vi "GetLibraryDependencies.vi"(11 "FileDependency":map{path, T1}(c390)) -> (2 "LibraryDependency":map{path, T3}(c390))   [LabVIEW 2020, in "DependencyViewer.lvlib"]
uses:
  DependencyViewer/DependencyViewer.lvlib
  LibraryDependentInfo.vi
  <vilib>/Utility/lvfile.llb/FT_FileTypes.ctl
  FileDependencyType.ctl
  <vilib>/Utility/miscctls.llb/LVMapReplaceAction.ctl
  <vilib>/Utility/lvfile.llb/NI_FileType.lvlib
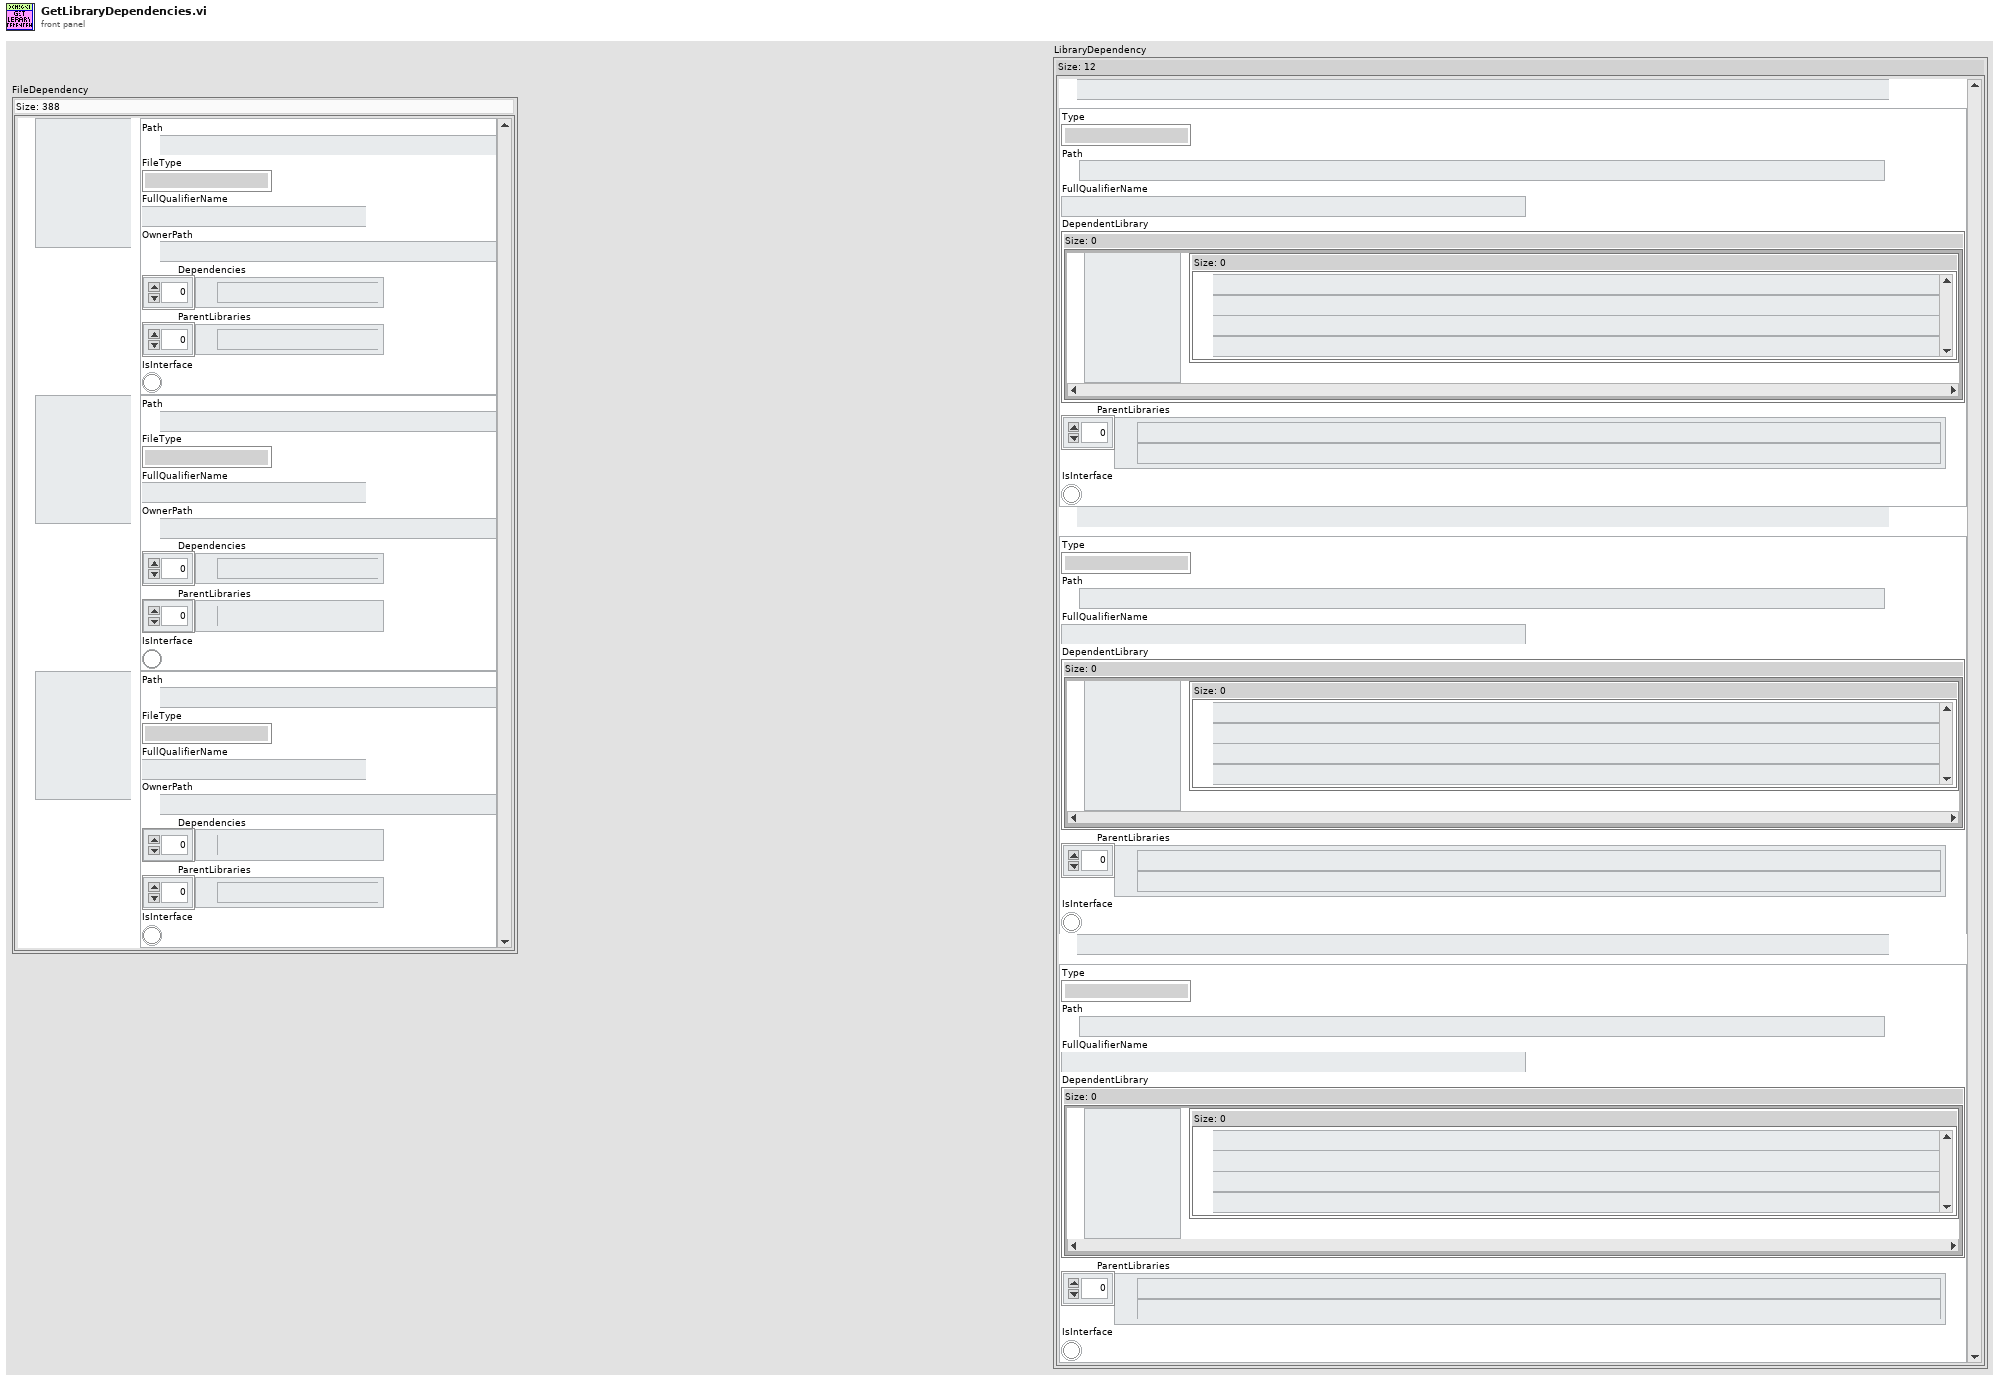
[diagram p1: front panel]
types:
  T1 = typedef "DependencyViewer.lvlib/FileDependencyType.ctl" = cluster{"Path":path, "FileType":T2, "FullQualifierName":string, "OwnerPath":path, "Dependencies":path[], "ParentLibraries":path[], "IsInterface":bool}
  T2 = typedef "NI_FileType.lvlib/FT_FileTypes.ctl" = enum32{"Invalid file/path", "Unknown type", "Instrument", "Control", "Polymorphic VI", "Project", "Library", "LVClass", "XControl", "XNode", "CIN", "Run-time menu", "Palette menu", "LLB", "Shortcut", "Directory", "Class Private Data Control", "Statechart", "MathScript .m file", "Ladder Diagram", "LVLibp"}
  T3 = typedef "DependencyViewer.lvlib/LibraryDependentInfo.vi" = cluster{"Type":T2, "Path":path, "FullQualifierName":string, "DependentLibrary":map{path, set{path}}, "ParentLibraries":path[], "IsInterface":bool}
  T4 = typedef "LVMapReplaceAction.ctl" = enum32{"Modify Entry only if found", "Add or Modify Entry", "Delete Entry"}
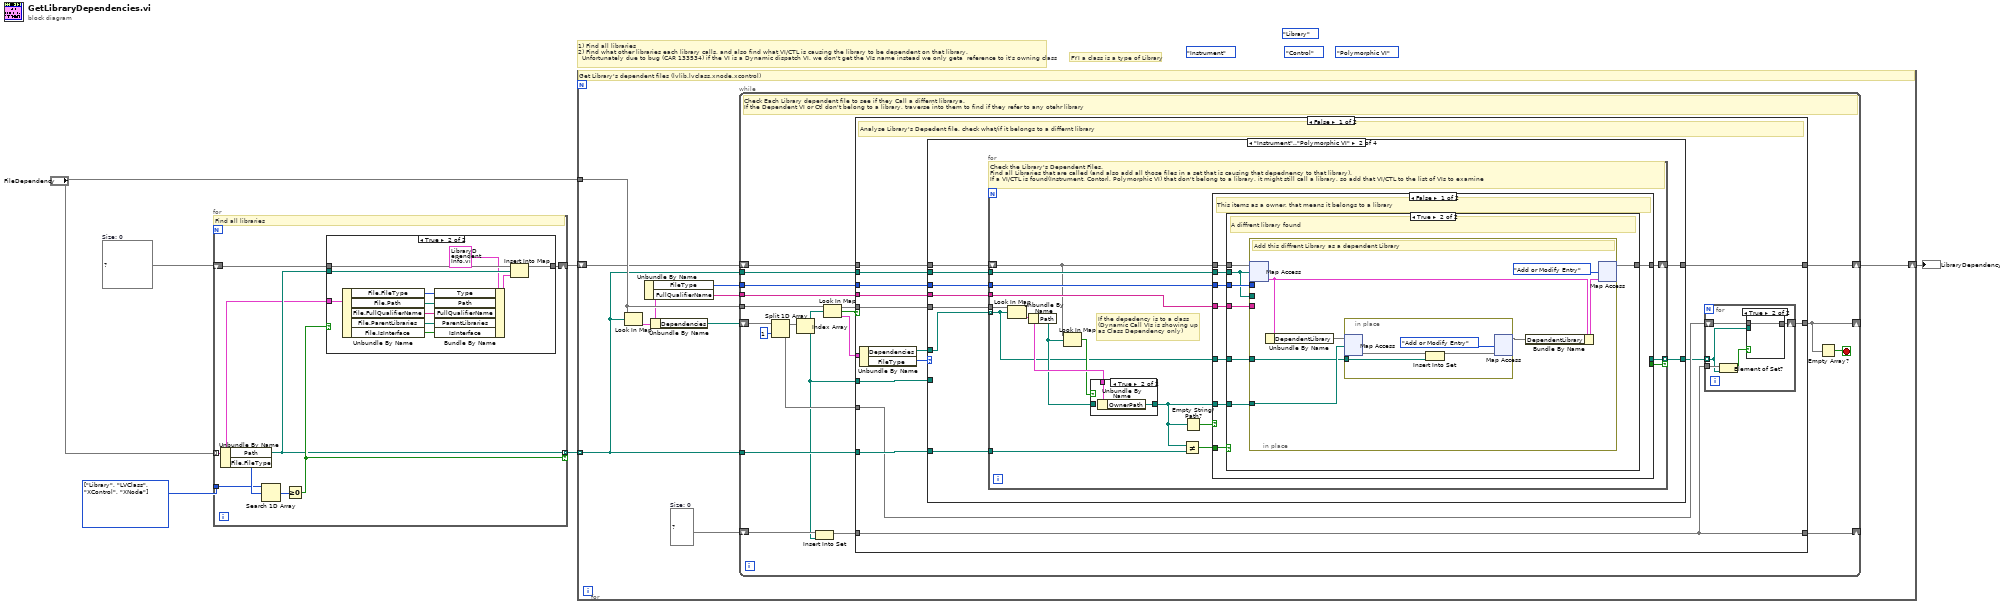
[diagram p0: block diagram]
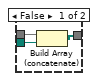
[diagram p2: hidden frame]
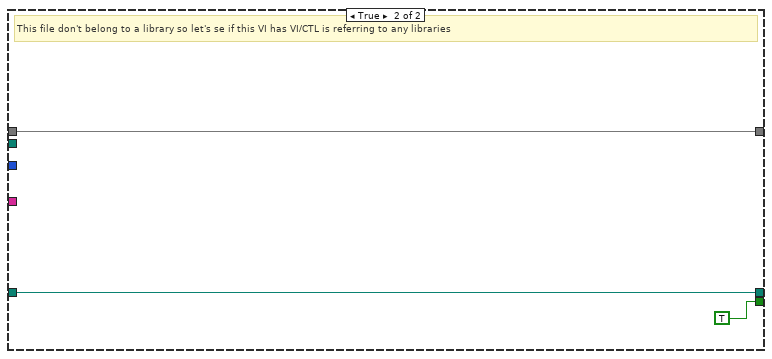
[diagram p5: hidden frame]
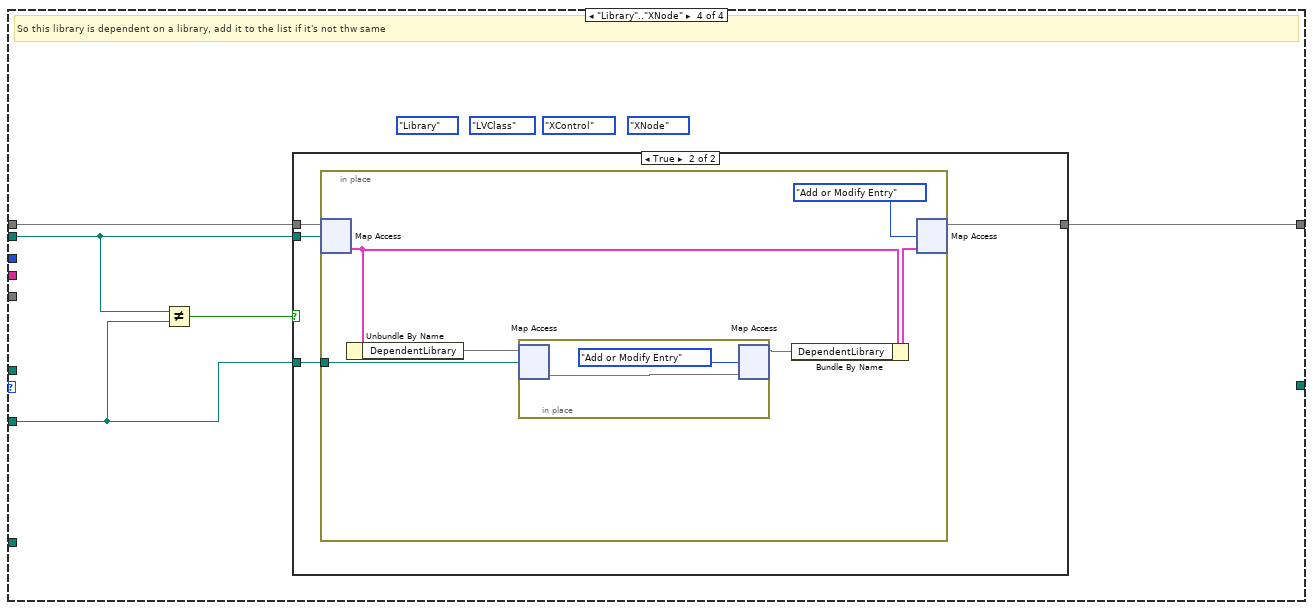
[diagram p8: hidden frame]
diagram:
  (unwired) FT_FileTypes."Library" ("FileType")
  (unwired) FT_FileTypes."Instrument" ("FileType")
  (unwired) FT_FileTypes."Control" ("FileType")
  (unwired) FT_FileTypes."Polymorphic VI" ("FileType")
  w5 = map{path, T3} {}  # Size: 0
  w3 = T2[] [enum."Library", enum."LVClass", enum."XControl", enum."XNode"] items=["Invalid file/path", "Unknown type", "Instrument", "Control", "Polymorphic VI", "Project", "Library", "LVClass", "XControl", "XNode", "CIN", "Run-time menu", "Palette menu", "LLB", "Shortcut", "Directory", "Class Private Data Control", "Statechart", "MathScript .m file", "Ladder Diagram", "LVLibp"] ("y")
  # "1) Find all libraries \n2) Find what other libraries each library calls, and also find what VI/CTL is causing the library to be dependent on that library.\n  Unfortunately due to bug (CAR 133534) if the VI is a Dynamic dispatch VI, we don't get the VIs name instead we only geta  reference to it's owning class"
  # "FYI a class is a type of Library"
  n1 = for {
    tunnel: "FileDependency" -> [w7] mode=indexing
    tunnel: [w8] -> w1 mode=indexing if=w11
    tunnel: w3 -> [w12]
    shift-right: [w9] -> w6
    shift-left: w5 -> [w10]
    # "Find all libraries"
    n2 = Unbundle By Name(w7) -> ("Path"=w8:path, "File.FileType"=w13:T2)
    n3 = Search 1D Array(1D array=w12, element=w13) -> (index of element=w14:i32)  [unwired: 1 in]
    n4 = Greater Or Equal To 0?(x=w14) -> (x >= 0?=w11:bool)
    n5 = case shown="True" w11 {
      tunnel: w10 -> [w15 w26]
      tunnel: [w15 w25] -> w9
      tunnel: w8 -> [_ w24]
      tunnel: w7 -> [_ w21]
      frame False {
      }
      frame True {
        n6 = Unbundle By Name(w21) -> ("File.FileType"=w20:T2, "File.Path"=w19:path, "File.FullQualifierName"=w18:string, "File.ParentLibraries"=w17:path[], "File.IsInterface"=w16:bool)
        n7 = Bundle By Name(cluster=T3 {"Type"=enum."Library", "Path"=path "", "FullQualifierName"="", "DependentLibrary"={}, "ParentLibraries"=[], "IsInterface"=FALSE} ("LibraryDependentInfo"), "Type"=w20, "Path"=w19, "FullQualifierName"=w18, "ParentLibraries"=w17, "IsInterface"=w16) -> (w22:T3)
        n8 = Insert Into Map(map in=w26, key=w24, value=w22) -> (map out=w25:map{path, T3})  [unwired: 2 out]
      }
    }
  }
  n9 = for {
    tunnel: w1 -> [w28] mode=indexing
    tunnel: "FileDependency" -> [w34]
    shift-right: [w32] -> w4
    shift-left: w6 -> [w33]
    w27 = set{path} {}  # Size: 0
    # "Get Library's dependent files (lvlib,lvclass,xnode,xcontrol)"
    n10 = Look In Map(map=w34, key=w28) -> (value=w31:T1)  [unwired: 1 in, 1 out]
    n11 = Unbundle By Name(w31) -> ("FileType"=w30:T2, "FullQualifierName"=w29:string)
    n12 = Unbundle By Name(w31) -> ("Dependencies"=w35:path[])
    n13 = while {
      tunnel: w34 -> [w53]
      tunnel: w28 -> [w52]
      shift-right: [w50] -> w32
      shift-left: w33 -> [w51]
      tunnel: w30 -> [w49]
      tunnel: w29 -> [w48]
      tunnel: w28 -> [w47]
      shift-right: [w43] -> _
      shift-left: w35 -> [w44]
      shift-right: [w36] -> _
      shift-left: w27 -> [w39]
      stop <- w42 stop-if-true
      # "Check Each Library dependent file to see if they Call a differnt librarya.\nIf the Dependent VI or Ctl don't belong to a library, traverse into them to find if they refer to any otehr library"
      n14 = Split 1D Array(array=w44, index=1) -> (first subarray=w45:path[], second subarray=w40:path[])
      n15 = Index Array(array=w45) -> (element=w38:path)  [unwired: 1 in]
      n16 = Insert Into Set(10:w38, 11:w39) -> (3:w37:set{path})  [unwired: 1 out]
      n17 = Look In Map(map=w53, key=w38) -> (key not found?=w41:bool, value=w54:T1)  [unwired: 1 in]
      n18 = case shown="False" w41 {
        tunnel: w54 -> [w69 _]
        tunnel: w53 -> [w68 _]
        tunnel: w52 -> [w66 _]
        tunnel: w51 -> [w65 w159]
        tunnel: [w64 w159] -> w50
        tunnel: w49 -> [w63 _]
        tunnel: w48 -> [w62 _]
        tunnel: w47 -> [w61 _]
        tunnel: w38 -> [w59 _]
        tunnel: [w57 w158] -> w43
        tunnel: w40 -> [w58 w158]
        tunnel: w37 -> [w55 w157]
        tunnel: [w55 w157] -> w36
        frame False {
          # "Analyse Library's Depedent file, check what/if it belongs to a differnt library"
          n19 = Unbundle By Name(w69) -> ("Dependencies"=w67:path[], "FileType"=w60:T2)
          n20 = case shown="\"Instrument\"..\"Polymorphic VI\"" w60 {
            tunnel: w68 -> [_ w88 _ _]
            tunnel: w67 -> [_ w87 _ _]
            tunnel: w66 -> [_ w86 _ _]
            tunnel: w65 -> [w79 w85 w138 w143]
            tunnel: [w79 w84 w138 w142] -> w64
            tunnel: w63 -> [_ w83 _ _]
            tunnel: w62 -> [_ w82 _ _]
            tunnel: w61 -> [_ w81 _ w140]
            tunnel: w59 -> [_ _ _ w141]
            tunnel: [_ w80 _ _] -> w56
            frame "Class Private Data Control" {
            }
            frame "Instrument".."Polymorphic VI" {
              n21 = for {
                tunnel: w88 -> [w104]
                tunnel: w87 -> [w93] mode=indexing
                tunnel: w86 -> [w103]
                shift-right: [w102] -> w84
                shift-left: w85 -> [w97]
                tunnel: w81 -> [w101]
                tunnel: w83 -> [w100]
                tunnel: w82 -> [w99]
                tunnel: [w90] -> w80 mode=indexing if=w89
                # "If the depedency is to a class\n(Dynamic Call VIs is showing up \nas Class Dependency only)"
                # "Check the Library's Dependent Files.\nFind all Libraries that are called (and also add all those files in a set that is causing that depednency to that library).\nIf a VI/CTL is found(Instrument, Contorl, Polymorphic VI) that don't belong to a library, it might still call a library, so add that VI/CTL to the list of VIs to examine"
                n22 = Look In Map(map=w104, key=w93) -> (value=w96:T1)  [unwired: 1 in, 1 out]
                n23 = Unbundle By Name(w96) -> ("Path"=w94:path)
                n24 = Look In Map(map=w97, key=w94) -> (key not found?=w95:bool)  [unwired: 1 in, 1 out]
                n25 = case shown="True" w95 {
                  tunnel: [w135 w137] -> w98
                  tunnel: w96 -> [_ w136]
                  tunnel: w94 -> [w135 _]
                  frame False {
                  }
                  frame True {
                    n26 = Unbundle By Name(w136) -> ("OwnerPath"=w137:path)
                  }
                }
                n27 = Not Equal?(x=w98, y=w103) -> (x != y?=w92:bool)
                n28 = Empty String/Path?(string/path=w98) -> (empty?=w91:bool)
                n29 = case shown="False" w91 {
                  tunnel: [w112 w134] -> w102
                  tunnel: w101 -> [w111 _]
                  tunnel: w100 -> [w110 _]
                  tunnel: w99 -> [w109 _]
                  tunnel: w98 -> [w108 _]
                  tunnel: w97 -> [w107 w134]
                  tunnel: w93 -> [w106 w133]
                  tunnel: w92 -> [w105 _]
                  tunnel: [_ w133] -> w90
                  tunnel: [_ TRUE] -> w89
                  frame False {
                    # "This items as a owner, that means it belongs to a library"
                    n30 = case shown="True" w105 {
                      tunnel: w107 -> [w113 w120]
                      tunnel: [w113 w114] -> w112
                      tunnel: w111 -> [_ w118]
                      tunnel: w110 -> [_ w119]
                      tunnel: w109 -> [_ w117]
                      tunnel: w108 -> [_ w116]
                      tunnel: w106 -> [_ w115]
                      frame False {
                        # "This VI/CTL belongs to this library, but we want to find other libraries this library is dependent on"
                      }
                      frame True {
                        # "A diffrent library found"
                        n31 = in-place {
                          in-place-border: w119 -> [_]
                          in-place-border: w118 -> [_]
                          in-place-border: w117 -> [_]
                          in-place-border: w116 -> [w122]
                          in-place-border: w115 -> [w121]
                          # "Add this diffrent Library as a dependent Library"
                          n32 = in-place-map #1(w120, w118) -> (w125:T3)  [unwired: 1 in, 1 out]
                          n33 = Unbundle By Name(w125) -> ("DependentLibrary"=w124:map{path, set{path}})
                          n34 = in-place {
                            in-place-border: w121 -> [w128]
                            n35 = in-place-map #2(w124, w122) -> (w130:set{path})  [unwired: 1 in, 1 out]
                            n36 = Insert Into Set(10:w128, 11:w130) -> (3:w129:set{path})  [unwired: 1 out]
                            n37 = in-place-map #2(w129, LVMapReplaceAction."Add or Modify Entry" ("action")) -> (w123:map{path, set{path}})  [unwired: 2 out]
                          }
                          n38 = Bundle By Name(cluster=w125, "DependentLibrary"=w123) -> (w126:T3)
                          n39 = in-place-map #1(w126, LVMapReplaceAction."Add or Modify Entry" ("action")) -> (w114:map{path, T3})  [unwired: 2 out]
                        }
                      }
                    }
                  }
                  frame True {
                    # "This file don't belong to a library so let's se if this VI has VI/CTL is referring to any libraries"
                  }
                }
              }
            }
            frame Default {
            }
            frame "Library".."XNode" {
              (unwired) FT_FileTypes."XNode" ("FileType")
              (unwired) FT_FileTypes."XControl" ("FileType")
              (unwired) FT_FileTypes."LVClass" ("FileType")
              (unwired) FT_FileTypes."Library" ("FileType")
              # "So this library is dependent on a library, add it to the list if it's not thw same"
              n40 = Not Equal?(x=w140, y=w141) -> (x != y?=w139:bool)
              n41 = case shown="True" w139 {
                tunnel: w143 -> [w144 w148]
                tunnel: [w144 w147] -> w142
                tunnel: w141 -> [_ w146]
                tunnel: w140 -> [_ w145]
                frame False {
                }
                frame True {
                  n42 = in-place {
                    in-place-border: w146 -> [w149]
                    n43 = in-place-map #3(w148, w145) -> (w152:T3)  [unwired: 1 in, 1 out]
                    n44 = Unbundle By Name(w152) -> ("DependentLibrary"=w151:map{path, set{path}})
                    n45 = in-place {
                      n46 = in-place-map #4(w151, w149) -> (w155:set{path})  [unwired: 1 in, 1 out]
                      n47 = in-place-map #4(w155, LVMapReplaceAction."Add or Modify Entry" ("action")) -> (w150:map{path, set{path}})  [unwired: 2 out]
                    }
                    n48 = Bundle By Name(cluster=w152, "DependentLibrary"=w150) -> (w153:T3)
                    n49 = in-place-map #3(w153, LVMapReplaceAction."Add or Modify Entry" ("action")) -> (w147:map{path, T3})  [unwired: 2 out]
                  }
                }
              }
            }
          }
          n50 = for {
            tunnel: w56 -> [w71] mode=indexing
            tunnel: w55 -> [w72]
            shift-right: [w73] -> w57
            shift-left: w58 -> [w74]
            n51 = Element of Set?(10:w71, 11:w72) -> (3:w70:bool)
            n52 = case shown="True" w70 {
              tunnel: w74 -> [w77 w78]
              tunnel: [w76 w78] -> w73
              tunnel: w71 -> [w75 _]
              frame False {
                n53 = Build Array (concatenate)(w77, w75) -> (w76:path[])
              }
              frame True {
              }
            }
          }
        }
        frame True {
          # "I guess this VI/CTL don't have any dependency"
        }
      }
      n54 = Empty Array?(array=w43) -> (empty?=w42:bool)
    }
  }
  "LibraryDependency" <- w4
